vi "Dev_interface.vi"() -> ()   [LabVIEW 2016]
uses:
  <vilib>/httpClient/LabVIEWHTTPClient.lvlib
  <vilib>/httpClient/ClientHandle.ctl
  <vilib>/httpClient/POSTBuffer.vi
  msg7171_linux.llb/send single message.vi
panel:
  out "MCC\nResp":string
  out "MCC Pwr":bool
  out "MCC Error":bool
  out "MCC_TurnTcOn_V":string
  out "MCC_TurnPumpOn_V":string
  out "MCC_TurnRoughOn_V":string
  out "MCC_TurnPurgeOn_V":string
  in  "MCC_SetRegen_V":u8(ring) items=["Abort Regen", "Start Full", "Start Fast", "Exit Standby", "Warm&Stop"]
  out "MCC 2nd stage Temp":string
  out "MCC 1st stage Temp":string
  out "MCCget_Ver_V":string
  out "MCC_RoughInterlock_V":string
  out "MCC_RegenSeq":string
  in  "Regen Standby Mode":string
  in  "Regen Repurge Time":string
  in  "Pumps per Compressor":string
  in  "Regen Rough Interlock":string
  in  "Regen Restart Temp":string
  in  "Regen Rt of Rise Cycles":string
  in  "Regen Rate of Rise":string
  in  "Regen Rough to Press":string
  in  "Regen Repurge Cycles":string
  in  "Regen Ext Purge Time":string
  in  "Regen Restart Delay":string
  out "MCC_DutyCycle":string
  out "MCC_TCpres":string
  in  "Get MCC":bool
  out "MCC_RegenTime":string
  in  "MCC_RoughInterlock":bool
  out "MCC_RegenError":string
  in  "MCC_SetRegen":bool
  in  "MCC_TurnTcOn":bool
  in  "MCC_TurnRoughOn":bool
  in  "MCC_TurnPurgeOn":bool
  in  "MCC_TurnPumpOn":bool
  in  "MCCset_2sgTemp":string
  in  "MCCset_1sgTemp":string
  in  "MCCget_Ver":bool
  in  "Get DIO":bool
  in  "Get PG":bool
  out "D In":bool[](array[boolean])
  in  "D Out":bool[](array[boolean])
  out "x/y":T1 {"Rouffing Pump" format="%#_6e"; "Chamber Pressure" format="%#_6e"; "Cryo Pump" format="%#_6e"}
  in  "exit":bool
  out "Waveform Chart":T2(graph)
  in  "Address":string="10.0.1.201"
  # "1\n2\n3\n4\n5\n6\n7\n8\n9\n10\n11\n12\n13\n14"
  # "1\n\n2\n\n3\n\n4\n\n5\n\n6"
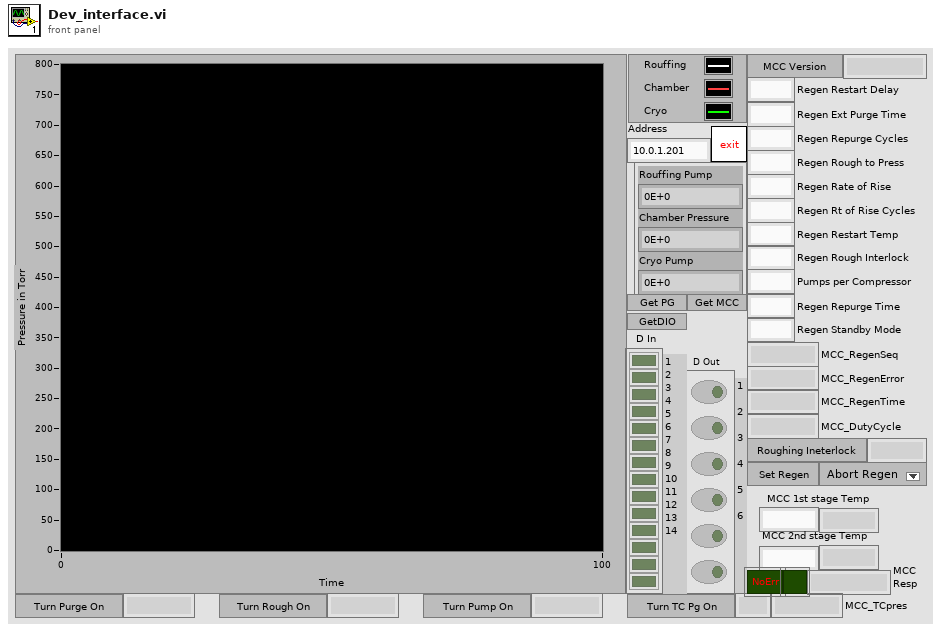
[diagram p1: front panel]
types:
  T1 = cluster{"Rouffing Pump":dbl, "Chamber Pressure":dbl, "Cryo Pump":dbl}
  T2 = cluster{"Pressure[0]":dbl, "Pressure[1]":dbl, "Pressure[2]":dbl}
  T3 = typedef "LabVIEWHTTPClient.lvlib/ClientHandle.ctl" = refnum<k1>
  T4 = cluster{"go":bool, "Http session":T3, "URL prefex":string}
  T5 = cluster{"Addr":i32[], "Kind":string[], "Pressure":dbl[]}
  T6 = cluster{"Error":bool, "PowerFailure":bool, "Data":string}
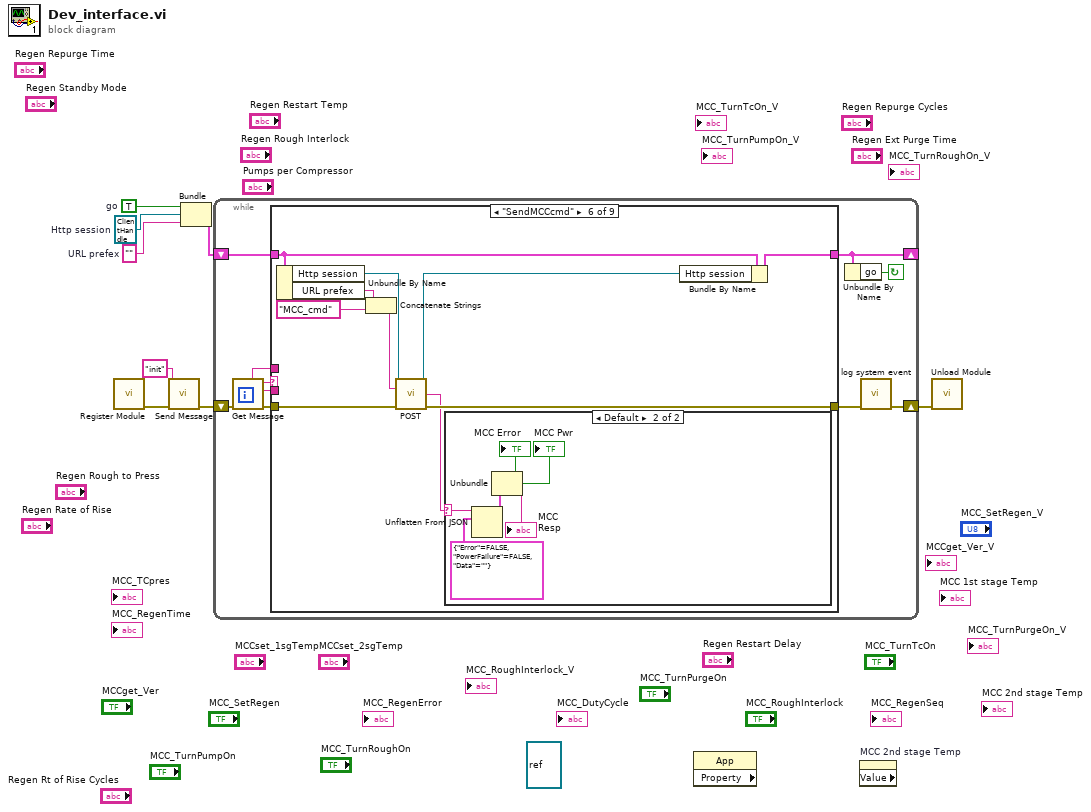
[diagram p0: block diagram]
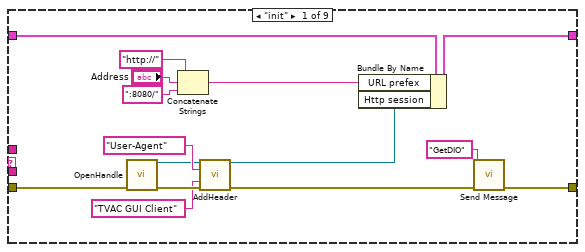
[diagram p2: hidden frame]
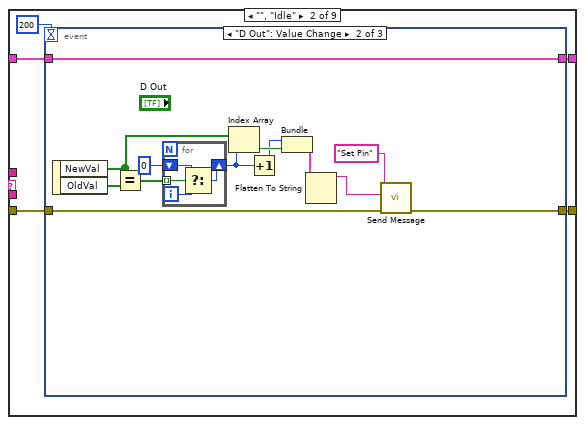
[diagram p3: hidden frame]
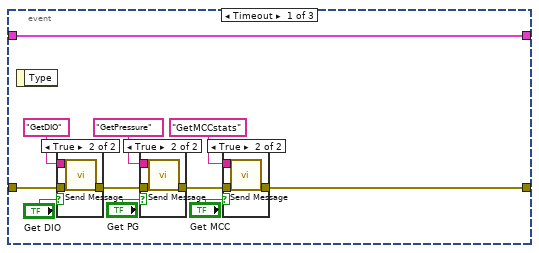
[diagram p4: hidden frame]
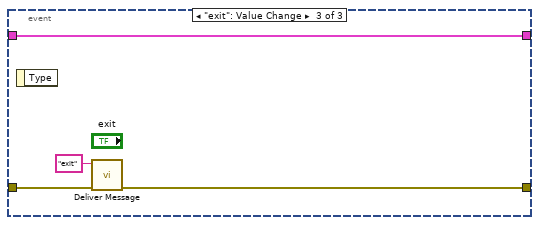
[diagram p8: hidden frame]
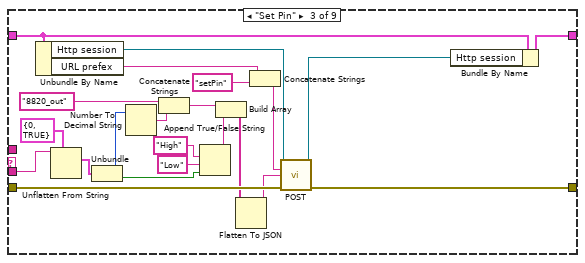
[diagram p9: hidden frame]
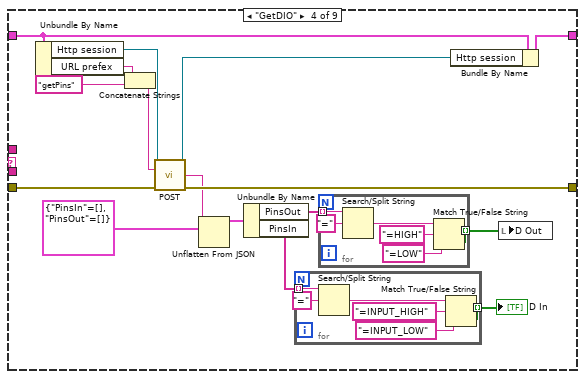
[diagram p10: hidden frame]
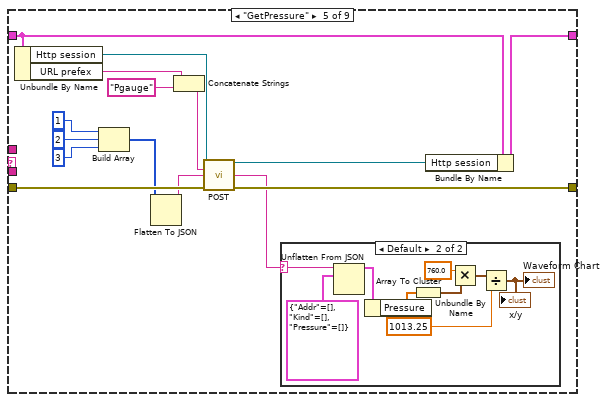
[diagram p11: hidden frame]
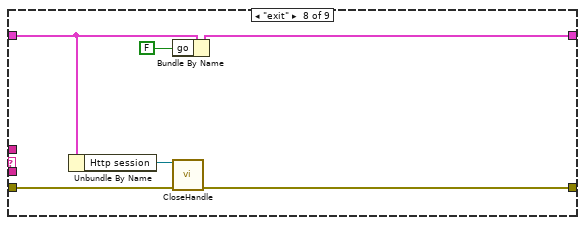
[diagram p15: hidden frame]
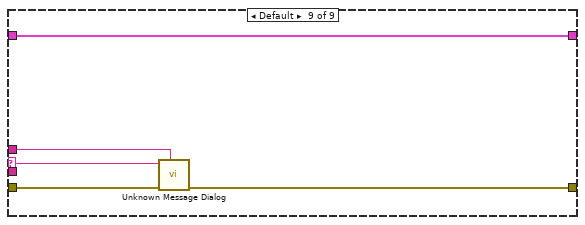
[diagram p16: hidden frame]
diagram:
  (unwired) refnum<vi> refnum ("reference")
  w4 = ""  # URL prefex
  w5 = T3 refnum  # Http session
  w6 = TRUE  # go
  n1 = call "Register Module.vi"() -> ("error out"=w2:errorcluster)  [unwired: 10 in, 1 out]
  n2 = call-poly "Send Message.vi"("error in (no error)"=w2, "event"="init") -> ("error out"=w1:errorcluster)  [unwired: 9 in]
  n3 = Bundle("go"=w6, "Http session"=w5, "URL prefex"=w4) -> (w8:T4)  [unwired: 1 in]
  n4 = while {
    shift-left: w8 -> [w15]
    shift-right: [w12] -> _
    shift-right: [w10] -> w7
    shift-left: w1 -> [w18]
    stop <- w11 continue-if-true
    n5 = call "Get Message.vi"("error in (no error)"=w18) -> ("error out"=w16:errorcluster, "event buffer"=w17:string, "event"=w14:string, "source"=w13:string)  [unwired: 7 in]
    n6 = case shown="\"SendMCCcmd\"" w14 {
      selector: w14 -> [_ _ _ _ _ _ _ _ w183]
      tunnel: [w24 w35 w97 w113 w145 w164 w174 w180 w185] -> w12
      tunnel: w15 -> [w33 w34 w96 w112 w143 w162 w174 w175 w185]
      tunnel: w17 -> [_ _ w86 _ _ _ _ _ _]
      tunnel: w16 -> [w28 w36 w99 w115 w147 w166 w173 w178 w184]
      tunnel: w13 -> [_ _ _ _ _ _ _ _ w182]
      tunnel: [w19 w38 w98 w114 w146 w165 w173 w177 w181] -> w9
      frame "init" {
        n7 = call <vilib>:"OpenHandle.vi"("error in (no error)"=w28) -> ("client handle out"=w29:T3, "error out"=w32:errorcluster)  [unwired: 13 in]
        n8 = Concatenate Strings("http://" ("url"), "Address", ":8080/" ("url")) -> (w23:string)
        n9 = call <vilib>:"AddHeader.vi"("client handle"=w29, "header"="User-Agent", "value"="TVAC GUI Client", "error in (no error)"=w32) -> ("client handle out"=w22:T3, "error out"=w20:errorcluster)  [unwired: 10 in]
        n10 = Bundle By Name(cluster=w33, "URL prefex"=w23, "Http session"=w22) -> (w24:T4)
        n11 = call-poly "Send Message.vi"("error in (no error)"=w20, "event"="GetDIO") -> ("error out"=w19:errorcluster)  [unwired: 9 in]
      }
      frame "", "Idle" {
        n12 = event shown="[1] \"D Out\": Value Change" {
          selector: _ -> [_ _ _]
          dyn-events: _ -> [_ _ _]
          timeout: 200 ("milliseconds to wait") -> [_ _ _]
          tunnel: w36 -> [w48 w65 w82]
          tunnel: [w39 w64 w81] -> w38
          tunnel: [w49 w74 w79] -> w35
          tunnel: w34 -> [w49 w74 w79]
          event Timeout {
            n13 = event-data() -> ()  [unwired: 1 in, 1 out]
            n14 = case shown="True" "Get DIO" {
              tunnel: w48 -> [w58 w61]
              tunnel: [w58 w60] -> w46
              tunnel: "GetDIO" ("event") -> [_ w59]
              frame False {
              }
              frame True {
                n15 = call-poly "Send Message.vi"("error in (no error)"=w61, "event"=w59) -> ("error out"=w60:errorcluster)  [unwired: 9 in]
              }
            }
            n16 = case shown="True" "Get PG" {
              tunnel: w46 -> [w54 w57]
              tunnel: [w54 w56] -> w40
              tunnel: "GetPressure" ("event") -> [_ w55]
              frame False {
              }
              frame True {
                n17 = call-poly "Send Message.vi"("error in (no error)"=w57, "event"=w55) -> ("error out"=w56:errorcluster)  [unwired: 9 in]
              }
            }
            n18 = case shown="True" "Get MCC" {
              tunnel: w40 -> [w50 w53]
              tunnel: [w50 w52] -> w39
              tunnel: "GetMCCstats" ("event") -> [_ w51]
              frame False {
              }
              frame True {
                n19 = call-poly "Send Message.vi"("error in (no error)"=w53, "event"=w51) -> ("error out"=w52:errorcluster)  [unwired: 9 in]
              }
            }
          }
          event "D Out": Value Change {
            n20 = event-data() -> ("NewVal"=w69:bool[], "OldVal"=w73:bool[])  [unwired: 1 in]
            n21 = Equal?(x=w69, y=w73) -> (x = y?=w72:bool[])
            n22 = for {
              tunnel: w72 -> [w78] mode=indexing
              shift-right: [w77] -> w70
              shift-left: 0 -> [w76]
              i -> [w75]
              n23 = Select(t=w76, s=w78, f=w75) -> (s? t:f=w77:i32)
            }
            n24 = Index Array(array=w69, index=w70) -> (element=w68:bool)
            n25 = Increment(x=w70) -> (x+1=w67:i32)
            n26 = Bundle(w67, "Boolean"=w68) -> (w63:cluster{i32, "Boolean":bool})  [unwired: 1 in]
            n27 = Flatten To String(anything=w63) -> (data string=w62:string)  [unwired: 3 in, 2 out]
            n28 = call-poly "Send Message.vi"("error in (no error)"=w65, "event buffer"=w62, "event"="Set Pin") -> ("error out"=w64:errorcluster)  [unwired: 8 in]
          }
          event "exit": Value Change {
            n29 = event-data() -> ()  [unwired: 1 in, 1 out]
            n30 = call "Deliver Message.vi"("error in (no error)"=w82, "event"="exit") -> ("error out"=w81:errorcluster)  [unwired: 9 in]
          }
        }
      }
      frame "Set Pin" {
        n31 = Unbundle By Name(w96) -> ("Http session"=w103:T3, "URL prefex"=w101:string)
        n32 = Unflatten From String(type=cluster{i32, bool} {0, TRUE}, binary string=w86) -> (value=w85:cluster{i32, bool})  [unwired: 3 in, 2 out]
        n33 = Unbundle(w85) -> (w84:i32, w83:bool)
        n34 = Number To Decimal String(number=w84) -> (decimal integer string=w88:string)  [unwired: 1 in]
        n35 = Concatenate Strings("8820_out" ("url"), w88) -> (w89:string)
        n36 = Append True/False String(1:w83, 2:"Low" ("url"), 3:"High" ("url")) -> (0:w92:string)  [unwired: 1 in]
        n37 = Build Array(w89, w92) -> (w94:string[])
        n38 = Flatten To JSON(anything=w94) -> (JSON string=w93:string)  [unwired: 2 in, 1 out]
        n39 = Concatenate Strings(w101, "setPin" ("url")) -> (w102:string)
        n40 = call-poly <vilib>:"POST.vi"("client handle"=w103, "url"=w102, "buffer"=w93, "error in (no error)"=w99) -> ("client handle out"=w104:T3, "error out"=w98:errorcluster)  [unwired: 8 in, 2 out]
        n41 = Bundle By Name(cluster=w96, "Http session"=w104) -> (w97:T4)
      }
      frame "GetDIO" {
        n42 = Unbundle By Name(w112) -> ("Http session"=w119:T3, "URL prefex"=w117:string)
        n43 = Concatenate Strings(w117, "getPins" ("url")) -> (w118:string)
        n44 = call-poly <vilib>:"POST.vi"("client handle"=w119, "url"=w118, "error in (no error)"=w115) -> ("client handle out"=w120:T3, "body"=w110:string, "error out"=w114:errorcluster)  [unwired: 9 in, 1 out]
        n45 = Unflatten From JSON(JSON string=w110, type and defaults=cluster{"PinsIn":string[], "PinsOut":string[]} {"PinsIn"=[], "PinsOut"=[]}) -> (value=w109:cluster{"PinsIn":string[], "PinsOut":string[]})  [unwired: 5 in, 1 out]
        n46 = Unbundle By Name(w109) -> ("PinsOut"=w108:string[], "PinsIn"=w106:string[])
        n47 = for {
          tunnel: w106 -> [w124] mode=indexing
          tunnel: [w122] -> w105 mode=indexing
          n48 = Search/Split String(string=w124, search string/char (-)="=") -> (match + rest of string=w121:string)  [unwired: 1 in, 2 out]
          n49 = Match True/False String(2:"=INPUT_LOW" ("false string"), 3:"=INPUT_HIGH" ("true string"), 4:w121) -> (0:w122:bool)  [unwired: 1 out]
        }
        "D In" <- w105
        n50 = for {
          tunnel: w108 -> [w130] mode=indexing
          tunnel: [w128] -> w107 mode=indexing
          n51 = Search/Split String(string=w130, search string/char (-)="=") -> (match + rest of string=w127:string)  [unwired: 1 in, 2 out]
          n52 = Match True/False String(2:"=LOW" ("false string"), 3:"=HIGH" ("true string"), 4:w127) -> (0:w128:bool)  [unwired: 1 out]
        }
        n53 = Bundle By Name(cluster=w112, "Http session"=w120) -> (w113:T4)
        n54 = local write "D Out"(w107) -> ()
      }
      frame "GetPressure" {
        n55 = Unbundle By Name(w143) -> ("Http session"=w142:T3, "URL prefex"=w140:string)
        n56 = Build Array(1, 2, 3) -> (w138:i32[])
        n57 = Flatten To JSON(anything=w138) -> (JSON string=w137:string)  [unwired: 2 in, 1 out]
        n58 = Concatenate Strings(w140, "Pgauge" ("url")) -> (w141:string)
        n59 = call-poly <vilib>:"POST.vi"("client handle"=w142, "url"=w141, "buffer"=w137, "error in (no error)"=w147) -> ("client handle out"=w144:T3, "body"=w136:string, "error out"=w146:errorcluster)  [unwired: 8 in, 1 out]
        n60 = case shown="Default" w136 {
          selector: w136 -> [_ w148]
          frame "" {
          }
          frame Default {
            n61 = Unflatten From JSON(JSON string=w148, type and defaults=T5 {"Addr"=[], "Kind"=[], "Pressure"=[]}) -> (value=w152:T5)  [unwired: 5 in, 1 out]
            n62 = Unbundle By Name(w152) -> ("Pressure"=w153:dbl[])
            n63 = Array To Cluster(array=w153) -> (cluster=w150:T2)
            n64 = Multiply(x=760.0, y=w150) -> (x*y=w154:T2)
            n65 = Divide(x=w154, y=1013.25) -> (x/y=→"Waveform Chart" →"x/y":T2)
          }
        }
        n66 = Bundle By Name(cluster=w143, "Http session"=w144) -> (w145:T4)
      }
      frame "SendMCCcmd" {
        n67 = Unbundle By Name(w162) -> ("Http session"=w161:T3, "URL prefex"=w159:string)
        n68 = Concatenate Strings(w159, "MCC_cmd" ("url")) -> (w160:string)
        n69 = call-poly <vilib>:"POST.vi"("client handle"=w161, "url"=w160, "error in (no error)"=w166) -> ("client handle out"=w163:T3, "body"=w157:string, "error out"=w165:errorcluster)  [unwired: 9 in, 1 out]
        n70 = case shown="Default" w157 {
          selector: w157 -> [_ w171]
          frame "" {
          }
          frame Default {
            n71 = Unflatten From JSON(JSON string=w171, type and defaults=T6 {"Error"=FALSE, "PowerFailure"=FALSE, "Data"=""}) -> (value=w170:T6)  [unwired: 5 in, 1 out]
            n72 = Unbundle(w170) -> ("Error"=→"MCC Error":bool, "PowerFailure"=→"MCC Pwr":bool, "Data"=→"MCC\nResp":string)
          }
        }
        n73 = Bundle By Name(cluster=w162, "Http session"=w163) -> (w164:T4)
      }
      frame "GetMCCstats" {
      }
      frame "exit" {
        n74 = Unbundle By Name(w175) -> ("Http session"=w176:T3)
        n75 = Bundle By Name(cluster=w175, "go"=FALSE ("Bundle Element")) -> (w180:T4)
        n76 = call <vilib>:"CloseHandle.vi"("client handle"=w176, "error in (no error)"=w178) -> ("error out"=w177:errorcluster)  [unwired: 13 in]
      }
      frame Default {
        n77 = call "Unknown Message Dialog.vi"("source"=w182, "error in (no error)"=w184, "event name"=w183) -> ("error out"=w181:errorcluster)  [unwired: 8 in]
      }
    }
    n78 = Unbundle By Name(w12) -> ("go"=w11:bool)
    n79 = call "log system event.vi"("error in (no error)"=w9) -> ("error out"=w10:errorcluster)  [unwired: 9 in, 1 out]
  }
  n80 = property class="App" props=[]() -> ()  [unwired: 2 in, 3 out]
  n81 = property on="MCC 2nd stage Temp" class="Str" props=["Value"]() -> ()  [unwired: 2 in, 3 out]
  n82 = call "Unload Module.vi"("error in (no error)"=w7) -> ()  [unwired: 10 in, 1 out]
